vi "Generate ReserveState ChangeEvent.vi"(8 "error in (no error)":errorcluster, 11 "SMO in":refnum<class "SMO.lvclass">) -> (0 "error out":errorcluster, 3 "SMO out":refnum<class "SMO.lvclass">)   [LabVIEW 2021, in "smo.lvlib" / "SMO.lvclass"]
uses:
  SMO.lvclass
  SMO.lvclass/SMO.ctl
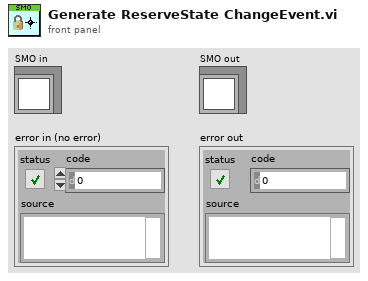
[diagram p1: front panel]
types:
  T1 = typedef "smo.lvlib/SMO.lvclass/Public Events.ctl" = cluster{"Error":refnum<user-event>, "State":refnum<user-event>, "Reserve State":refnum<user-event>}
  T2 = typedef "smo.lvlib/SMO.lvclass/Accessibility--Cluster.ctl" = cluster{"Lock Key":string, "Reserve State":T3}
  T3 = typedef "smo.lvlib/SMO.lvclass/Reserve State--Enum.ctl" = enum16{"Unreserved", "Reserved", "Self-locked"}
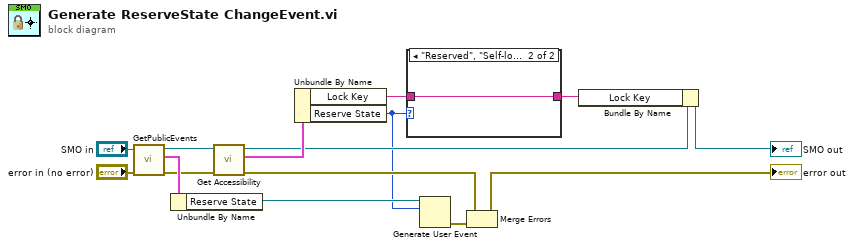
[diagram p0: block diagram]
diagram:
  n1 = call "GetPublicEvents.vi"("error in (no error)"="error in (no error)", "SMO"="SMO in") -> ("error out"=w8:errorcluster, "Public Events"=w12:T1, "SMO out"=w9:refnum<class "SMO.lvclass">)  [unwired: 7 in]
  n2 = Unbundle By Name(w12) -> ("Reserve State"=w13:refnum<user-event>)
  n3 = call "Get Accessibility.vi"("error in (no error)"=w8, "SMO"=w9) -> ("error out"=w7:errorcluster, "Accessibility"=w6:T2, "SMO out"=w5:refnum<class "SMO.lvclass">)  [unwired: 7 in]
  n4 = Unbundle By Name(w6) -> ("Lock Key"=w2:string, "Reserve State"=w3:T3)
  n5 = case shown="\"Reserved\", \"Self-locked\"" w3 {
    tunnel: w2 -> [_ w16]
    tunnel: [_ w16] -> w1
    frame "Unreserved" {
    }
    frame "Reserved", "Self-locked" {
    }
  }
  n6 = Generate User Event(user event=w13, event data cluster=w3) -> (error out=w14:errorcluster)  [unwired: 2 in, 1 out]
  n7 = Merge Errors(w7, w14) -> (→"error out":errorcluster)
  n8 = Bundle By Name(cluster=w5, "Lock Key"=w1) -> (→"SMO out":refnum<class "SMO.lvclass">)
